vi "Clear Multicolumn Listbox.vi"(8 "error in":errorcluster, 11 "MulticolumnListbox in":refnum<vi>) -> (0 "error out":errorcluster)   [LabVIEW 2017, in "DTacq Plot Display Library.lvlib"]
doc: "Clears all text and colour from a multicolumn listbox."
uses:
  DTacq Plot Display Library.lvlib
  <vilib>/Utility/miscctls.llb/LVRowAndColumnTypeDef.ctl
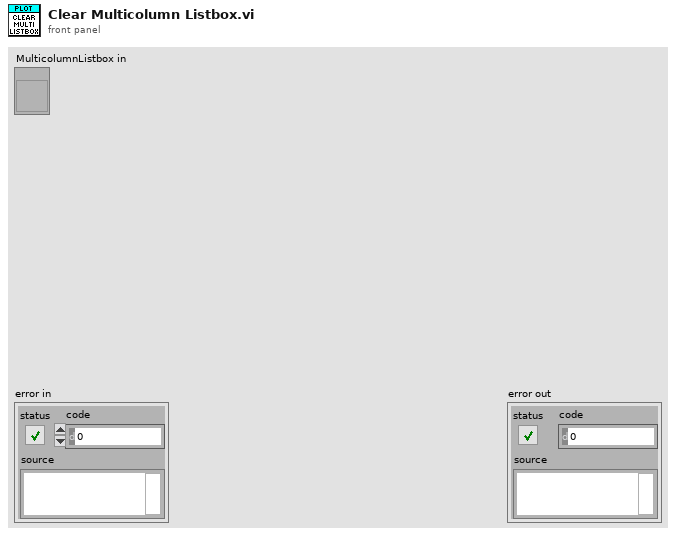
[diagram p1: front panel]
types:
  T1 = typedef "LVRowAndColumnTypeDef.ctl" = cluster{"Row":i32, "Column":i32}
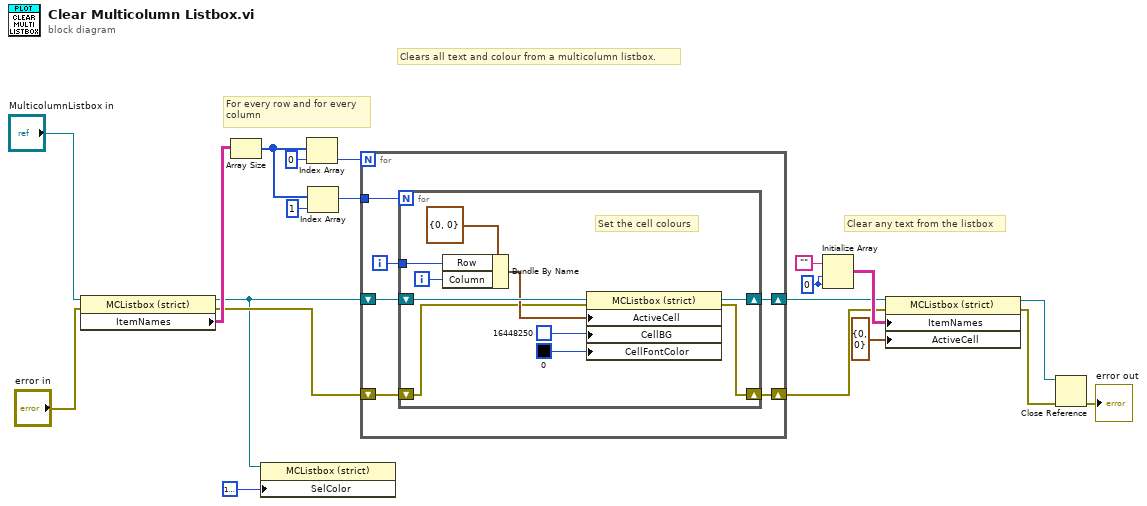
[diagram p0: block diagram]
diagram:
  w8 = 0 ("dimension size")
  # "Clear any text from the listbox"
  # "For every row and for every\ncolumn"
  # "Clears all text and colour from a multicolumn listbox."
  n1 = property class="MCListbox (strict)"(reference="MulticolumnListbox in", error in="error in") -> (reference out=w3:refnum<vi>, error out=w13:errorcluster, "ItemNames"=w15:string[][])
  n2 = Array Size(array=w15) -> (size(s)=w18:i32[])
  n3 = property class="MCListbox (strict)"(reference=w3, "SelColor"=u32 16777222) -> ()  [unwired: 1 in, 2 out]
  n4 = Index Array(array=w18, index=0) -> (element=w17:i32)
  n5 = Index Array(array=w18, index=1) -> (element=w20:i32)
  n6 = for {
    N: w17 -> [_]
    tunnel: w20 -> [w25]
    shift-right: [w22] -> w7
    shift-left: w3 -> [w26]
    shift-right: [w21] -> w4
    shift-left: w13 -> [w23]
    i -> [w24]
    n7 = for {
      N: w25 -> [_]
      tunnel: w24 -> [w33]
      shift-right: [w28] -> w22
      shift-left: w26 -> [w36]
      shift-right: [w27] -> w21
      shift-left: w23 -> [w29]
      i -> [w32]
      # "Set the cell colours"
      n8 = Bundle By Name(cluster=T1 {"Row"=0, "Column"=0} ("Active Cell:Active Cell"), "Row"=w33, "Column"=w32) -> (w34:T1)
      n9 = property class="MCListbox (strict)"(reference=w36, error in=w29, "ActiveCell"=w34, "CellBG"=u32 16448250 ("Plot Colour Box 2"), "CellFontColor"=u32 0 ("Plot Colour Box 2")) -> (reference out=w28:refnum<vi>, error out=w27:errorcluster)
    }
  }
  n10 = Initialize Array("", w8, w8) -> (w10:string[][])
  n11 = property class="MCListbox (strict)"(reference=w7, error in=w4, "ItemNames"=w10, "ActiveCell"=T1 {"Row"=0, "Column"=0} ("Active Cell:Active Cell")) -> (reference out=w6:refnum<vi>, error out=w5:errorcluster)
  n12 = Close Reference(reference=w6, error in (no error)=w5) -> (error out=→"error out":errorcluster)
